vi "Write Callchain.vi"(8 "error in (no error)":errorcluster, 10 "Callchain":string, 11 "LogRecord in":refnum<class "LogRecord.lvclass">) -> (0 "error out":errorcluster, 3 "LogRecord out":refnum<class "LogRecord.lvclass">)   [LabVIEW 2016, in "hse-logger.lvlib" / "LogRecord.lvclass"]
uses:
  LogRecord.lvclass
  LogRecord.lvclass/LogRecord.ctl
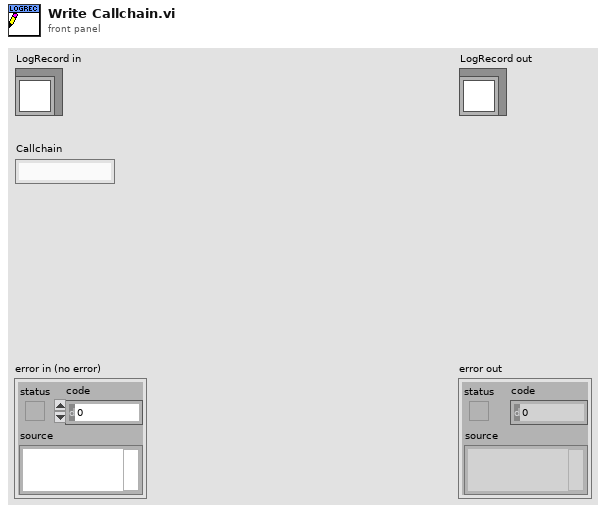
[diagram p1: front panel]
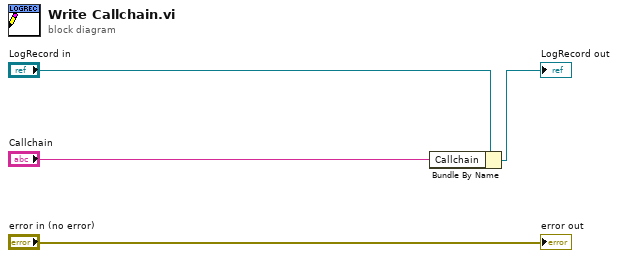
[diagram p0: block diagram]
diagram:
  n1 = Bundle By Name(cluster="LogRecord in", "Callchain"="Callchain") -> (→"LogRecord out":refnum<class "LogRecord.lvclass">)
  "error out" <- "error in (no error)"
